vi "Nod_Head.vi"(0 "error in":errorcluster, 3 "node":string) -> (1 "error out":errorcluster)   [LabVIEW 2010]
doc: "This will nod the head."
uses:
  ROS/MessageBuilding/std_msgs/subs/boolScalar.vi
  ROS/Code/SubVIs/_ROSDirection.ctl
  ROS/Code/Console/Servers/ServerSubs/TopicDef.ctl
panel:
  in  "State":bool=TRUE
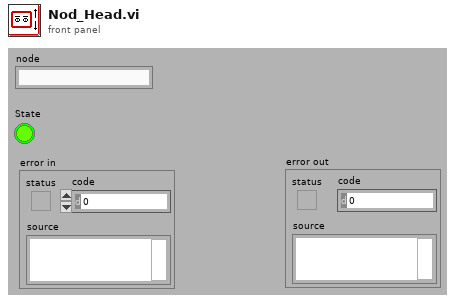
[diagram p1: front panel]
types:
  T1 = typedef "TopicDef.ctl" = cluster{"Topic":string, "Type":string, "Action":T2, "Update (ms)":u16, "write queue":u16}
  T2 = typedef "_ROSDirection.ctl" = enum16{"Node", "Publisher", "Subscriber", "Service Client"}
  T3 = typedef "_ROSControl.ctl" = cluster{"topic port":u16, "Node":string, "topic":string, "type":string, "node port":u32, "error ":errorcluster, "Direction":T2, "APIs":string[], "Update (ms)":u16, "write queue":u16}
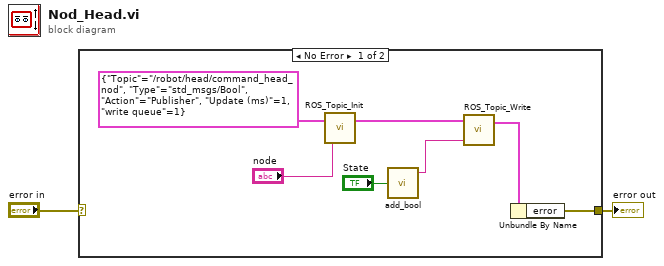
[diagram p0: block diagram]
diagram:
  n1 = case shown="No Error" "error in" {
    selector: "error in" -> [_ w10]
    tunnel: [w7 w10] -> w2
    frame No Error {
      n2 = call "ROS_Topic_Init.vi"("node"="node", "Definitions"=T1 {"Topic"="/robot/head/command_head_nod", "Type"="std_msgs/Bool", "Action"=enum."Publisher", "Update (ms)"=1, "write queue"=1}) -> ("ROS out"=w9:T3)  [unwired: 1 in]
      n3 = call-poly "add_bool.vi"("Boolean"="State") -> ("msg out"=w5:string)  [unwired: 4 in]
      n4 = call "ROS_Topic_Write.vi"("Msg in"=w5, "ROS in"=w9) -> ("ROS out"=w8:T3)  [unwired: 2 in]
      n5 = Unbundle By Name(w8) -> ("error"=w7:errorcluster)
    }
    frame Error {
    }
  }
  "error out" <- w2
